vi "Thorlabs-PMT Safety Check.vi"(8 "error in (no error)":errorcluster) -> (0 "error out":errorcluster, 3 "Stop":bool, 4 "User message":string)   [LabVIEW 2020]
uses:
  _Globals/Global Controls.vi
  ECU_SDK/ThorECU.lvlib
panel:
  # "Checks PMT A and B for saturation and if so, disables the saturated PMT(s) and sets gain to 1"
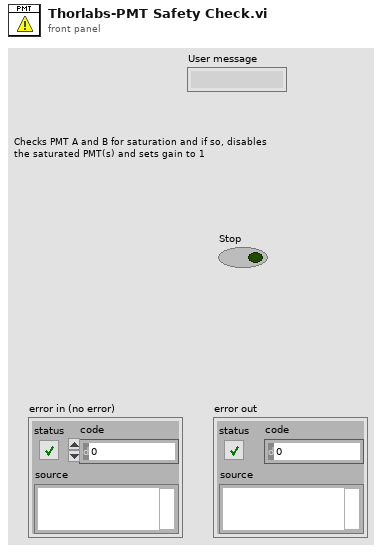
[diagram p1: front panel]
types:
  T1 = typedef "Tweezertron Ctrl Refs.ctl" = cluster{"LSM Settings":refnum<vi>, "iFlex Control":refnum<vi>, "PIFOC Settings":refnum<vi>, "PinSelector":refnum<vi>, "Manlight Controls":refnum<vi>, "Exp Params":refnum<vi>, "Image Thresholds":refnum<vi>, "RevFrame":refnum<vi>, "Spots":refnum<vi>}
  T2 = typedef "Confocal Controls.ctl" = cluster{"Channel Selection":enum32{"A", "B", "AB"}, "Pixel Count":cluster{"Pixels in X":u32, "Pixels in Y":u32}, "Field Size":dbl, "Frames":u8, "Averaging":bool, "Alignment":dbl, "Scan Mode":bool, "Gain":cluster{"Gain A":u8, "Gain B":u8}, "Enable PMTs":cluster{"A":bool, "B":bool}, "Voltage Range":cluster{"Range A":u16, "Range B":u16}, "Multi Frame Count":dbl, "Trigger Mode":dbl, "Real Time Averaging":bool, "PFOV":dbl, "MicronsPerPx":dbl}
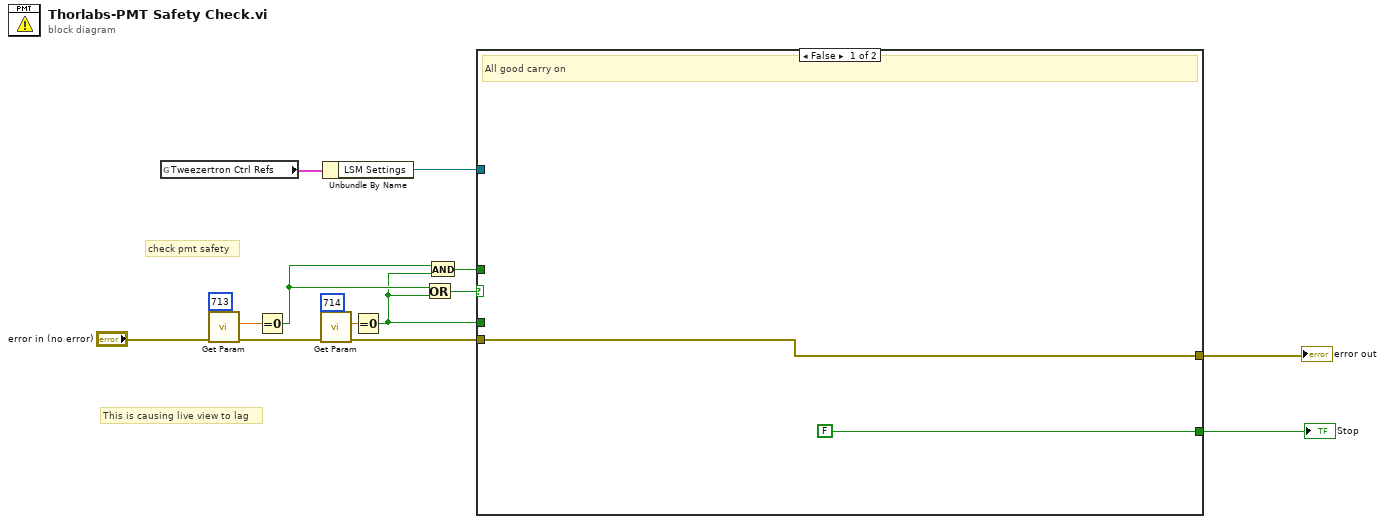
[diagram p0: block diagram]
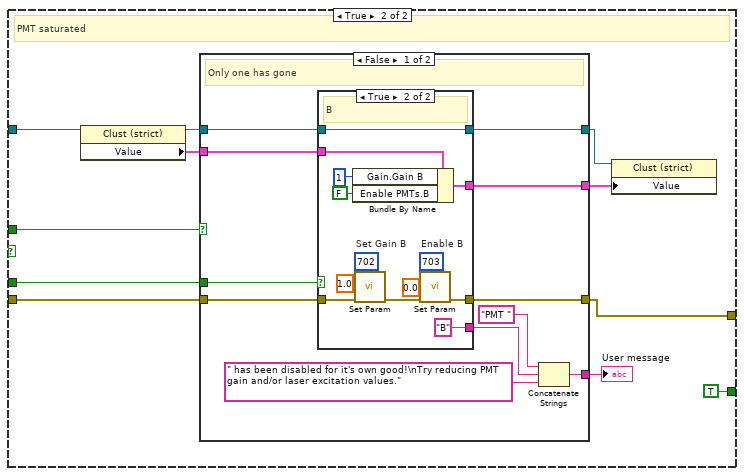
[diagram p2: hidden frame]
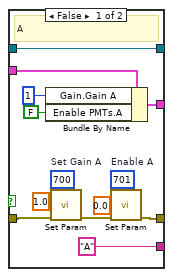
[diagram p3: hidden frame]
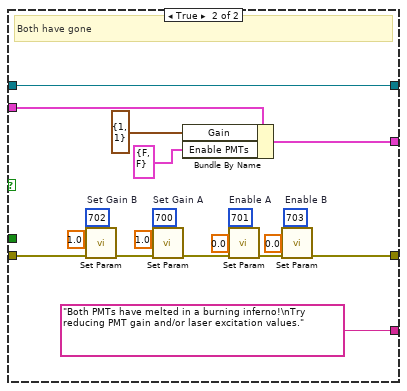
[diagram p4: hidden frame]
diagram:
  # "This is causing live view to lag"
  # "check pmt safety"
  n1 = global read "Global Controls.vi" "Tweezertron Ctrl Refs"() -> (w3:T1)
  n2 = call "Get Param.vi"("error in (no error)"="error in (no error)", "paramID"=713) -> ("error out"=w8:errorcluster, "param out"=w1:dbl)  [unwired: 7 in, 1 out]
  n3 = Equal To 0?(x=w1) -> (x = 0?=w6:bool)
  n4 = call "Get Param.vi"("error in (no error)"=w8, "paramID"=714) -> ("error out"=w12:errorcluster, "param out"=w11:dbl)  [unwired: 7 in, 1 out]
  n5 = Unbundle By Name(w3) -> ("LSM Settings"=w2:refnum<vi>)
  n6 = Equal To 0?(x=w11) -> (x = 0?=w5:bool)
  n7 = Or(x=w6, y=w5) -> (x .or. y?=w14:bool)
  n8 = And(x=w6, y=w5) -> (x .and. y?=w4:bool)
  n9 = case shown="False" w14 {
    tunnel: w12 -> [w17 w28]
    tunnel: [w17 w21] -> w7
    tunnel: [FALSE ("Yeah, whatever") TRUE ("Yeah, whatever")] -> w13
    tunnel: w5 -> [_ w26]
    tunnel: w4 -> [_ w25]
    tunnel: w2 -> [_ w18]
    frame False {
      # "All good carry on"
    }
    frame True {
      # "PMT saturated"
      n10 = property on="Property Node" class="Clust (strict)"(reference=w18) -> (reference out=w24:refnum<vi>, "Value"=w27:T2)  [unwired: 1 in, 1 out]
      n11 = case shown="False" w25 {
        tunnel: w26 -> [w37 _]
        tunnel: [w35 "Both PMTs have melted in a burning inferno!\nTry reducing PMT gain and/or laser excitation values."] -> w19
        tunnel: w28 -> [w34 w73]
        tunnel: [w33 w71] -> w21
        tunnel: w27 -> [w32 w70]
        tunnel: [w31 w68] -> w22
        tunnel: w24 -> [w30 w66]
        tunnel: [w29 w66] -> w23
        frame False {
          # "Only one has gone"
          n12 = case shown="True" w37 {
            tunnel: ["A" ("string") "B" ("string")] -> w36
            tunnel: w34 -> [w43 w56]
            tunnel: [w44 w59] -> w33
            tunnel: w32 -> [w47 w60]
            tunnel: [w45 w61] -> w31
            tunnel: w30 -> [w41 w54]
            tunnel: [w41 w54] -> w29
            frame False {
              w50 = 700  # Set Gain A
              w48 = 701  # Enable A
              # "A"
              n13 = Bundle By Name(cluster=w47, "Gain.Gain A"=u8 1 ("Gain A"), "Enable PMTs.A"=FALSE) -> (w45:T2)
              n14 = call "Set Param.vi"("error in (no error)"=w43, "param"=1.0, "paramID"=w50) -> ("error out"=w42:errorcluster)  [unwired: 7 in, 1 out]
              n15 = call "Set Param.vi"("error in (no error)"=w42, "param"=0.0, "paramID"=w48) -> ("error out"=w44:errorcluster)  [unwired: 7 in, 1 out]
            }
            frame True {
              w58 = 702  # Set Gain B
              w63 = 703  # Enable B
              # "B"
              n16 = Bundle By Name(cluster=w60, "Gain.Gain B"=u8 1 ("Gain A"), "Enable PMTs.B"=FALSE) -> (w61:T2)
              n17 = call "Set Param.vi"("error in (no error)"=w56, "param"=1.0, "paramID"=w58) -> ("error out"=w55:errorcluster)  [unwired: 7 in, 1 out]
              n18 = call "Set Param.vi"("error in (no error)"=w55, "param"=0.0, "paramID"=w63) -> ("error out"=w59:errorcluster)  [unwired: 7 in, 1 out]
            }
          }
          n19 = Concatenate Strings("PMT " ("string"), w36, " has been disabled for it's own good!\nTry reducing PMT gain and/or laser excitation values." ("Message")) -> (w35:string)
        }
        frame True {
          w76 = 700  # Set Gain A
          w78 = 702  # Set Gain B
          w82 = 701  # Enable A
          w80 = 703  # Enable B
          # "Both have gone"
          n20 = call "Set Param.vi"("error in (no error)"=w73, "param"=1.0, "paramID"=w78) -> ("error out"=w74:errorcluster)  [unwired: 7 in, 1 out]
          n21 = call "Set Param.vi"("error in (no error)"=w74, "param"=1.0, "paramID"=w76) -> ("error out"=w72:errorcluster)  [unwired: 7 in, 1 out]
          n22 = Bundle By Name(cluster=w70, "Gain"=cluster{"Gain A":u8, "Gain B":u8} {"Gain A"=1, "Gain B"=1} ("Value"), "Enable PMTs"=cluster{bool, bool} {FALSE, FALSE}) -> (w68:T2)
          n23 = call "Set Param.vi"("error in (no error)"=w72, "param"=0.0, "paramID"=w82) -> ("error out"=w84:errorcluster)  [unwired: 7 in, 1 out]
          n24 = call "Set Param.vi"("error in (no error)"=w84, "param"=0.0, "paramID"=w80) -> ("error out"=w71:errorcluster)  [unwired: 7 in, 1 out]
        }
      }
      "User message" <- w19
      n25 = property class="Clust (strict)"(reference=w23, "Value"=w22) -> ()  [unwired: 1 in, 2 out]
    }
  }
  "Stop" <- w13
  "error out" <- w7
